vi "Multichannel demo2016.vi"() -> ()   [LabVIEW 2016]
uses:
  D/0_Perovskite tandem solar cell_Monash/Monash Center Lab trainings/Laser room/Development package/Labview/V12/base_xml.llb/Type Descriptor Enumeration__ogtk.ctl
panel:
  out "Plugged channels":i32[](array[numeric])
  in  "VSCAN Parameters":T1={"tb"=5e-05, "vs_initial "=TRUE, "Voltage_step"=0.0, "Scans"=[{" vs_initial "=FALSE, "Voltage_step"=0.1, "Scan_Rate"=0.1}, {" vs_initial "=FALSE, "Voltage_step"=-0.2, "Scan_Rate"=0.1}, {" vs_initial "=FALSE, "Voltage_step"=0.0, "Scan_Rate"=0.1}], "Scan_number"=2, "N_Cycles"=0, "Record_every_dE"=0.01, "Begin_measuring_I"=0.5, "End_measuring_I"=0.75, "I_Range"=12, "E_Range"=3, "Bandwidth"=5, "em"=1, "ce"=0} {"tb" min=5e-05 max=1 format="%^_3e"; "ce" items=["Standard", "CE to ground"]; "End_measuring_I" min=0 max=1 format="%.2f"; "Begin_measuring_I" min=0 max=1 format="%.2f"; "Voltage_step" min=-10 max=10 format="%^_3e"; "N_Cycles" min=0 max=1000000; "Scan_number" min=0 max=98; "Scans"."Scan_Rate" min=1e-05 max=10 format="%^_3e"; "Scans"."Voltage_step" format="%^_3e"; "E_Range" items=["±2.5V", "±5V", "±10V", "Auto"]; "Bandwidth" items=["1"=1, "2"=2, "3"=3, "4"=4, "5"=5, "6"=6, "7"=7, "8"=8, "9"=9]; "Record_every_dE" format="%^_3e"; "I_Range" items=["1pA", "1nA", "10nA", "100nA", "1µA", "10µA", "100µA", "1mA", "10mA", "100mA", "1A", "Booster", "Auto"]}
  out "BW disabled ranges":i32[](array[numeric])
  out "current disabled ranges":i32[](array[numeric])
  out "Channel information":T2 {"NbAmp" min=5 max=7; "LcBoard" min=5 max=7; "AmpCode" min=5 max=7}
  out "Number of available Channels":u32
  out "ID":i32
  in  "First Channels":u8(ring) items=["1", "2", "3", "4", "5", "6", "7", "8", "9", "10", "11", "12", "13", "14", "15", "16"]
  out "Device Code":i32
  out "TDeviceINfo":T3 {"nb of slots" min=5 max=7}
  in  "IP adress":string="192.109.209.229"
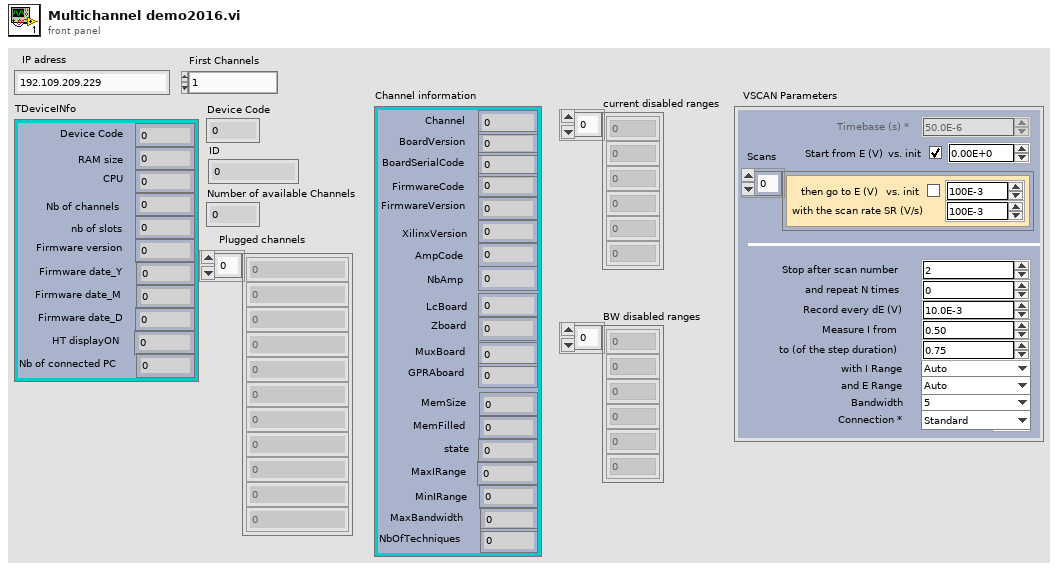
[diagram p1: front panel]
types:
  T1 = cluster{"tb":sgl, "vs_initial ":bool, "Voltage_step":sgl, "Scans":cluster{" vs_initial ":bool, "Voltage_step":sgl, "Scan_Rate":sgl}[], "Scan_number":i32, "N_Cycles":i32, "Record_every_dE":sgl, "Begin_measuring_I":sgl, "End_measuring_I":sgl, "I_Range":u16, "E_Range":u16, "Bandwidth":u16, "em":u16, "ce":u16}
  T2 = cluster{"Channel":i32, "BoardVersion":i32, "BoardSerialCode":i32, "FirmwareCode":i32, "FirmwareVersion":i32, "XilinxVersion":i32, "AmpCode":i32, "NbAmp":i32, "LcBoard":i32, "Zboard":i32, "MuxBoard":i32, "GPRAboard":i32, "MemSize":i32, "MemFilled":i32, "state":i32, "MaxIRange":i32, "MinIRange":i32, "MaxBandwidth":i32, "NbOfTechniques":i32}
  T3 = cluster{"Device Code":i32, "RAM size":i32, "CPU":i32, "Nb of channels":i32, "nb of slots":i32, "Firmware version":i32, "Firmware date_Y":i32, "Firmware date_M":i32, "Firmware date_D":i32, "HT displayON":i32, "Nb of connected PC":i32}
  T4 = typedef "Type Descriptor Enumeration__ogtk.ctl" = enum8{"<Null>", "I8", "I16", "I32", "I64", "U8", "U16", "U32", "U64", "SGL", "DBL", "EXT", "CSG", "CDB", "CXT", "0x0F", "0x10", "0x11", "0x12", "0x13", "0x14", "Enum U8", "Enum U16", "Enum U32", "Enum U64", "SGL PQ", "DBL PQ", "EXT PQ", "CSG PQ", "CDB PQ", "CXT PQ", "0x1F", "0x20", "Boolean", "0x22", "0x23", "0x24", "0x25", "0x26", "0x27", "0x28", "0x29", "0x2A", "0x2B", "0x2C", "0x2D", "0x2E", "0x2F", "String", "0x31", "Path", "Pict", "0x34", "0x35", "0x36", "DAQ", "0x38", "0x39", "0x3A", "0x3B", "0x3C", "0x3D", "0x3E", "0x3F", "Array", "0x41", "0x42", "0x43", "0x44", "0x45", "0x46", "0x47", "0x48", "0x49", "0x4A", "0x4B", "0x4C", "0x4D", "0x4E", "0x4F", "Cluster", "0x51", "0x52", "Variant", "Waveform", "0x55", "0x56", "0x57", "0x58", "0x59", "0x5A", "0x5B", "0x5C", "0x5D", "0x5E", "0x5F", "0x60", "0x61", "0x62", "0x63", "0x64", "0x65", "0x66", "0x67", "0x68", "0x69", "0x6A", "0x6B", "0x6C", "0x6D", "0x6E", "0x6F", "Refnum"}
  T5 = cluster{"Data Type":T4, "Format String":string}[]
  T6 = cluster{" vs_initial ":bool, "Voltage_step":sgl, "Scan_Rate":sgl}[]
  T7 = cluster{" vs_initial ":bool, "Voltage_step":sgl, "Scan_Rate":sgl}
  T8 = cluster{"Label":string, "type":i32, "valeur":u32, "index":i32}[]
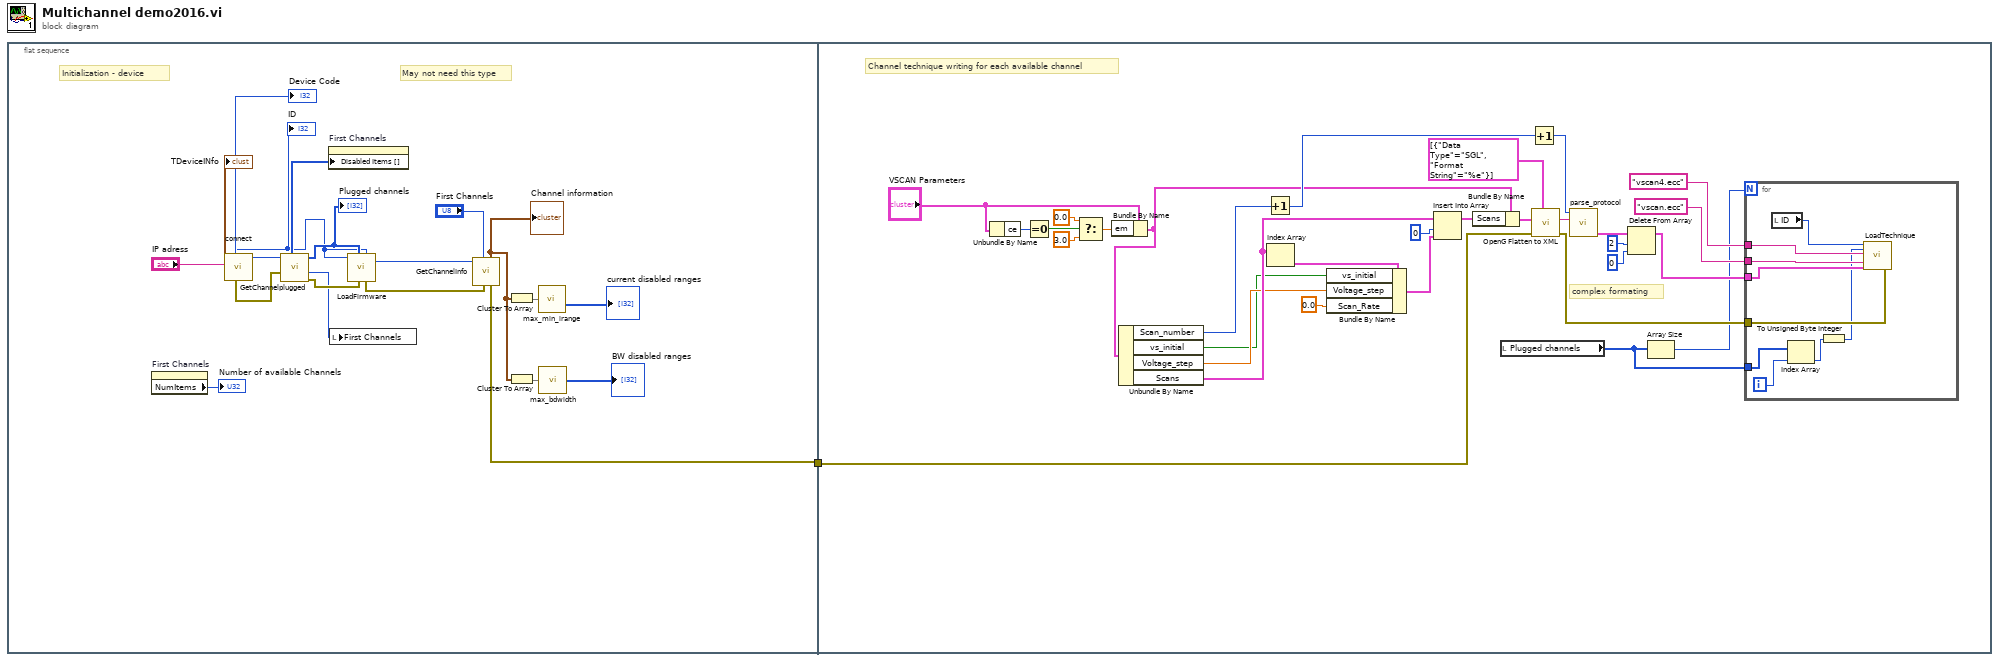
[diagram p0: block diagram]
diagram:
  n1 = flat-sequence {
    tunnel: [w2] -> w1
    tunnel: w1 -> [w20]
    frame #0 {
      # "May not need this type"
      # "Initialization - device"
      n2 = property on="First Channels" class="Ring (strict)"() -> ("NumItems"=→"Number of available Channels":u32)  [unwired: 2 in, 2 out]
      n3 = call "connect.vi"("IP"="IP adress") -> ("error out"=w17:errorcluster, "Device Code"=→"Device Code":i32, "TDeviceINfo"=→"TDeviceINfo":T3, "ID"=w7:i32)  [unwired: 7 in]
      "ID" <- w7
      n4 = call "GetChannelplugged.vi"("error in (no error)"=w17, "ID"=w7) -> ("error out"=w16:errorcluster, "First channel"=w8:i32, "Disabled channels"=w13:i32[], "Plugged channels"=w18:i32[])  [unwired: 6 in]
      "Plugged channels" <- w18
      n5 = property on="First Channels" class="Ring (strict)"("Disabled Items []"=w13) -> ()  [unwired: 2 in, 2 out]
      n6 = local write "First Channels"(w8) -> ()
      n7 = call "LoadFirmware.vi"("error in (no error)"=w16, "Channels"=w18, "ID"=w7) -> ("error out"=w6:errorcluster)  [unwired: 7 in, 1 out]
      n8 = call "GetChannelInfo.vi"("error in (no error)"=w6, "Channel"="First Channels", "ID"=w7) -> ("error out"=w2:errorcluster, "Channel information"=w9:T2)  [unwired: 7 in]
      "Channel information" <- w9
      n9 = Cluster To Array(cluster=w9) -> (array=w11:i32[])
      n10 = Cluster To Array(cluster=w9) -> (array=w10:i32[])
      n11 = call "max_min_irange.vi"("resources"=w11) -> ("disabled ranges"=→"current disabled ranges":i32[])
      n12 = call "max_bdwidth.vi"("resources"=w10) -> ("disabled ranges"=→"BW disabled ranges":i32[])
    }
    frame #1 {
      # "complex formating"
      # "Channel technique writing for each available channel"
      n13 = Unbundle By Name("VSCAN Parameters") -> ("ce"=w28:u16)
      n14 = Equal To 0?(x=w28) -> (x = 0?=w27:bool)
      n15 = Select(t=0.0, s=w27, f=3.0) -> (s? t:f=w30:dbl)
      n16 = Bundle By Name(cluster="VSCAN Parameters", "em"=w30) -> (w24:T1)
      n17 = Unbundle By Name(w24) -> ("Scan_number"=w33:i32, "vs_initial"=w38:bool, "Voltage_step"=w39:sgl, "Scans"=w42:T6)
      n18 = Increment(x=w33) -> (x+1=w34:i32)
      n19 = Index Array(array=w42) -> (element=w36:T7)  [unwired: 1 in]
      n20 = Bundle By Name(cluster=w36, "vs_initial"=w38, "Voltage_step"=w39, "Scan_Rate"=sgl 0.0) -> (w40:T7)
      n21 = Insert Into Array(array=w42, index=0 ("indice"), new element=w40) -> (w43:T6)
      n22 = Bundle By Name(cluster=w24, "Scans"=w43) -> (w35:T1)
      n23 = local read "Plugged channels"() -> (w21:i32[])
      n24 = Increment(x=w34) -> (x+1=w32:i32)
      n25 = call "OpenG Flatten to XML.vi"("Type Formats (default)"=T5 [{"Data Type"=enum."SGL", "Format String"="%e"}] ("Type Formats"), "error in (no error)"=w20, "LabVIEW Data"=w35) -> ("error out"=w47:errorcluster, "XML String"=w48:string)  [unwired: 7 in]
      n26 = call "parse_protocol.vi"("XML String In"=w48, "index array"=w32) -> ("Params Values"=w44:T8)  [unwired: 7 in]
      n27 = Delete From Array(array=w44, length=2 ("longueur"), index=0 ("indice")) -> (array with subset deleted=w23:T8)  [unwired: 1 out]
      n28 = Array Size(array=w21) -> (size(s)=w22:i32)
      n29 = for {
        N: w22 -> [_]
        tunnel: "vscan.ecc" ("FName") -> [w59]
        tunnel: w47 -> [w58]
        tunnel: "vscan4.ecc" ("FName") -> [w57]
        tunnel: w23 -> [w55]
        tunnel: w21 -> [w54]
        i -> [w53]
        n30 = local read "ID"() -> (w56:i32)
        n31 = Index Array(array=w54, index=w53) -> (element=w52:i32)
        n32 = To Unsigned Byte Integer(number=w52) -> (unsigned 8bit integer=w51:u8)
        n33 = call "LoadTechnique.vi"("ID"=w56, "Selected Channel"=w51, "FName4"=w57, "FName"=w59, "Protocol Parameters"=w55, "error in (no error)"=w58) -> ()  [unwired: 13 in, 1 out]
      }
    }
  }
